vi "Asylum_Interpolation.vi"(0 "X":dbl[](array[numeric]), 1 "Y":dbl[](array[numeric]), 2 "V":dbl[](array[numeric]), 3 "Interpolation":dbl format="%#_13g") -> (7 "X":dbl[](array[numeric]), 8 "Y":dbl[](array[numeric]), 9 "V":dbl[](array[numeric]))   [LabVIEW 2020]
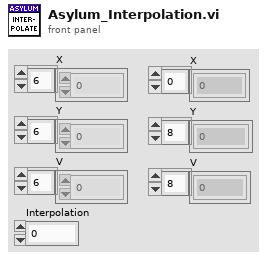
[diagram p1: front panel]
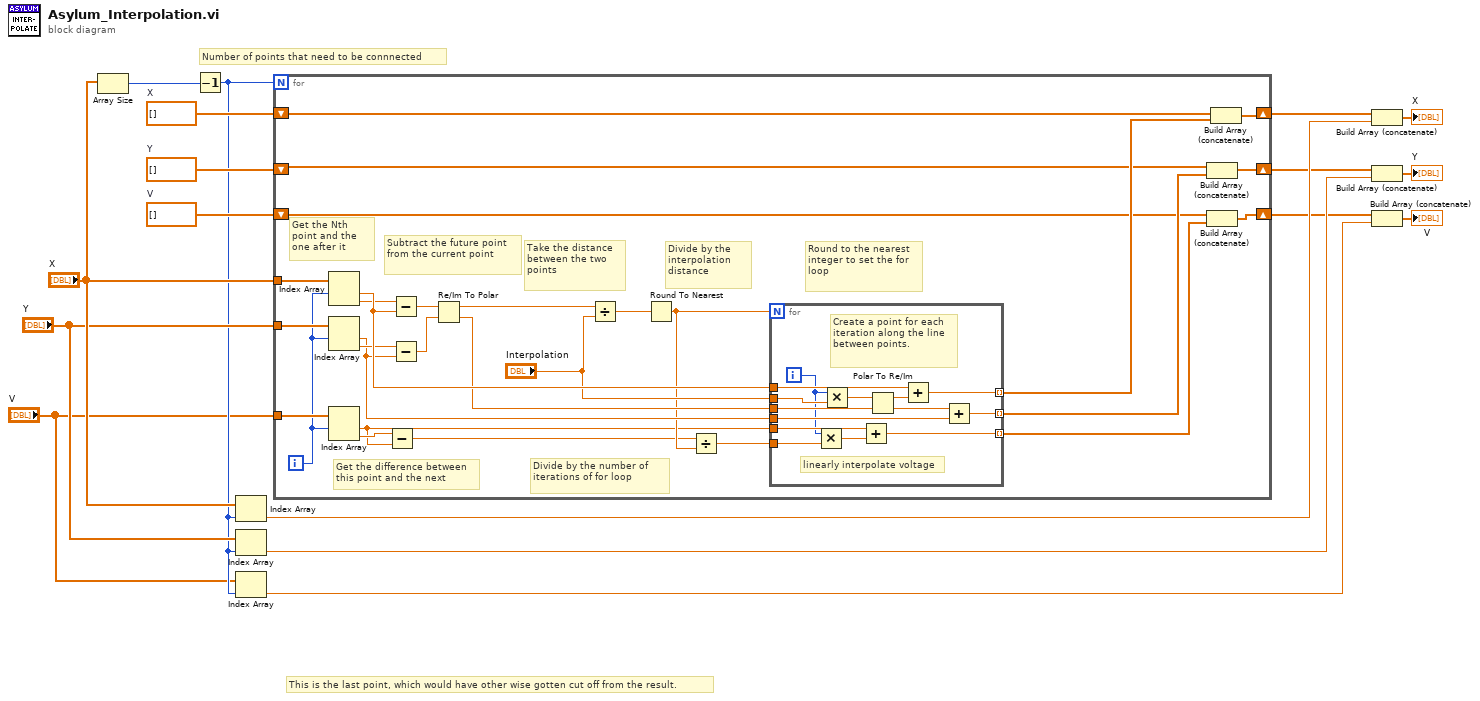
[diagram p0: block diagram]
diagram:
  w6 = dbl[] []  # V
  w12 = dbl[] []  # Y
  w13 = dbl[] []  # X
  # "This is the last point, which would have other wise gotten cut off from the result."
  # "Number of points that need to be connnected"
  n1 = Array Size(array="X") -> (size(s)=w14:i32)
  n2 = Decrement(x=w14) -> (x-1=w4:i32)
  n3 = Index Array(array="X", index=w4) -> (element=w16:dbl)
  n4 = Index Array(array="Y", index=w4) -> (element=w9:dbl)
  n5 = Index Array(array="V", index=w4) -> (element=w2:dbl)
  n6 = for {
    N: w4 -> [_]
    tunnel: "X" -> [w45]
    shift-right: [w40] -> w17
    shift-left: w13 -> [w39]
    tunnel: "Y" -> [w38]
    shift-right: [w32] -> w10
    shift-left: w12 -> [w31]
    tunnel: "V" -> [w28]
    shift-right: [w19] -> w5
    shift-left: w6 -> [w20]
    i -> [w27]
    # "Divide by the number of iterations of for loop"
    # "Get the difference between this point and the next"
    # "Subtract the future point from the current point"
    # "Get the Nth point and the one after it"
    # "Round to the nearest integer to set the for loop"
    # "Divide by the interpolation distance"
    # "Take the distance between the two points"
    n7 = Index Array(array=w45, index #1=w27) -> (element #1=w42:dbl, element #2=w41:dbl)  [unwired: 1 in]
    n8 = Index Array(array=w38, index #1=w27) -> (element #1=w34:dbl, element #2=w36:dbl)  [unwired: 1 in]
    n9 = Index Array(array=w28, index #1=w27) -> (element #1=w22:dbl, element #2=w26:dbl)  [unwired: 1 in]
    n10 = Subtract(x=w26, y=w22) -> (x-y=w24:dbl)
    n11 = Subtract(x=w41, y=w42) -> (x-y=w37:dbl)
    n12 = Subtract(x=w36, y=w34) -> (x-y=w35:dbl)
    n13 = Re/Im To Polar(2:w35, 3:w37) -> (0:w30:dbl, 1:w44:dbl)
    n14 = Divide(x=w44, y="Interpolation") -> (x/y=w43:dbl)
    n15 = Round To Nearest(number=w43) -> (nearest integer value=w25:dbl)
    n16 = Divide(x=w24, y=w25) -> (x/y=w23:dbl)
    n17 = for {
      N: w25 -> [_]
      tunnel: w42 -> [w51]
      tunnel: "Interpolation" -> [w52]
      tunnel: w30 -> [w58]
      tunnel: w34 -> [w54]
      tunnel: [w56] -> w21 mode=indexing
      tunnel: [w55] -> w33 mode=indexing
      tunnel: w23 -> [w46]
      tunnel: w22 -> [w49]
      tunnel: [w48] -> w18 mode=indexing
      i -> [w47]
      # "linearly interpolate voltage"
      # "Create a point for each iteration along the line between points."
      n18 = Multiply(x=w47, y=w46) -> (x*y=w50:dbl)
      n19 = Multiply(x=w47, y=w52) -> (x*y=w59:dbl)
      n20 = Add(x=w49, y=w50) -> (x+y=w48:dbl)
      n21 = Polar To Re/Im(2:w58, 3:w59) -> (0:w53:dbl, 1:w57:dbl)
      n22 = Add(x=w51, y=w57) -> (x+y=w55:dbl)
      n23 = Add(x=w53, y=w54) -> (x+y=w56:dbl)
    }
    n24 = Build Array (concatenate)(w31, w21) -> (w32:dbl[])
    n25 = Build Array (concatenate)(w20, w18) -> (w19:dbl[])
    n26 = Build Array (concatenate)(w39, w33) -> (w40:dbl[])
  }
  n27 = Build Array (concatenate)(w17, w16) -> (→"X":dbl[])
  n28 = Build Array (concatenate)(w10, w9) -> (→"Y":dbl[])
  n29 = Build Array (concatenate)(w5, w2) -> (→"V":dbl[])
